vi "xeva-main.vi"() -> ()   [LabVIEW 2015]
uses:
  <vilib>/Xenics Infrared Solutions/Xeneth LabVIEW API/Xeneth.lvlib
panel:
  in  "stop-acquisition":bool
  out "Histogram":T1(graph)={"X Values"=[381.555, 1026.665, 1671.775, 2316.885, 2961.995, 3607.105, 4252.215, 4897.325, 5542.435, 6187.545, 6832.655, 7477.765, 8122.875, 8767.985, 9413.095, 10058.205, 10703.315, 11348.425, 11993.535, 12638.645, 13283.755, 13928.865, 14573.975, 15219.085, 15864.195, 16509.305, 17154.415, 17799.525, 18444.635, 19089.745, 19734.855, 20379.965, 21025.075, 21670.185, 22315.295, 22960.405, 23605.515, 24250.625, 24895.735, 25540.845, 26185.955, 26831.065, 27476.175, 28121.285, 28766.395, 29411.505, 30056.615, 30701.725, 31346.835, 31991.945, 32637.055, 33282.165, 33927.275, 34572.385, 35217.495, 35862.605, 36507.715, 37152.825, 37797.935, 38443.045, 39088.155, 39733.265, 40378.375, 41023.485, 41668.595, 42313.705, 42958.815, 43603.925, 44249.035, 44894.145, 45539.255, 46184.365, 46829.475, 47474.585, 48119.695, 48764.805, 49409.915, 50055.025, 50700.135, 51345.245, 51990.355, 52635.465, 53280.575, 53925.685, 54570.795, 55215.905, 55861.015, 56506.125, 57151.235, 57796.345, 58441.455, 59086.565, 59731.675, 60376.785, 61021.895, 61667.005, 62312.115, 62957.225, 63602.335, 64247.445], "Histogram: h(x)"=[235, 173, 0, 115, 75, 0, 36, 38, 0, 21, 0, 14, 13, 0, 16, 28, 0, 49, 0, 91, 118, 0, 184, 328, 0, 436, 626, 0, 854, 0, 1158, 1443, 0, 1891, 2217, 0, 2808, 0, 3354, 3711, 0, 4252, 4588, 0, 4786, 0, 4898, 4792, 0, 4596, 4273, 0, 3970, 3545, 0, 3221, 0, 3015, 2668, 0, 2533, 2324, 0, 2214, 0, 2124, 1991, 0, 1897, 1839, 0, 1906, 0, 1861, 1832, 0, 1883, 1841, 0, 1844, 1875, 0, 1813, 0, 1765, 1729, 0, 1611, 1524, 0, 1290, 0, 1154, 968, 0, 749, 585, 0, 491, 313]}
  out "data":u16[][](array[numeric])
  out "error out":errorcluster
  out "temperature reached":bool
  in  "stop-parameter-read":bool
  out "cooling":bool
  out "temperature":bool
  in  "temperature / °C":dbl=-10.0
  out "Parameter":T2 {"time" format="%#.2g"}
  out "integration time":bool
  in  "integration time / s":dbl=1.0
  out "xeva initialized":bool
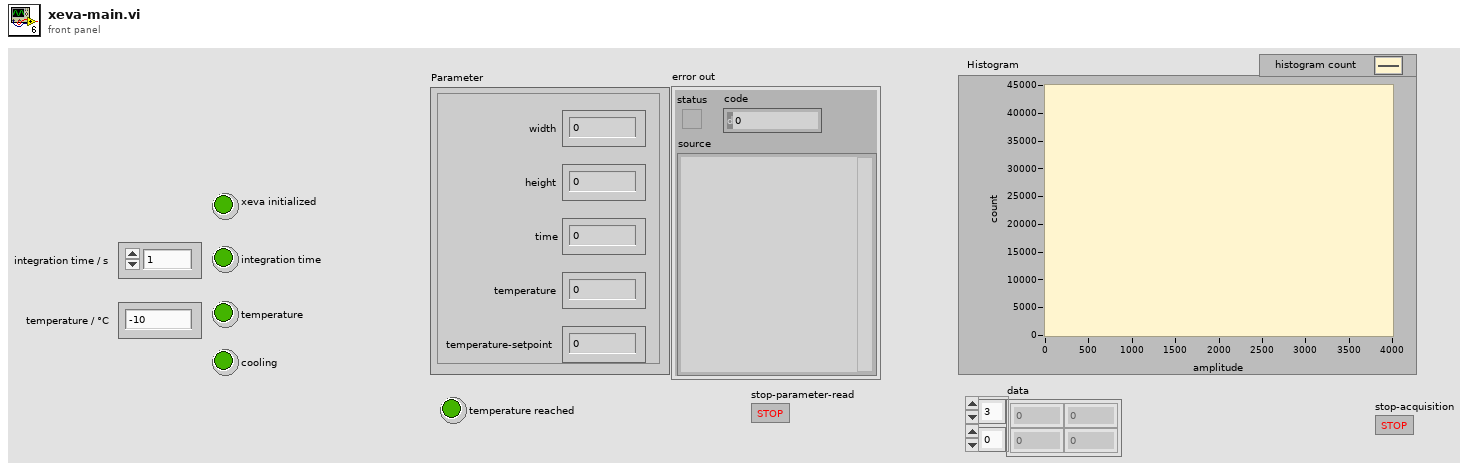
[diagram p1: front panel]
types:
  T1 = cluster{"X Values":dbl[], "Histogram: h(x)":i32[]}
  T2 = cluster{"width":u32, "height":u32, "time":dbl, "temperature":dbl, "temperature-setpoint":dbl}
  T3 = typedef "Xeneth.lvlib/Camara.ctl" = refnum<k1>
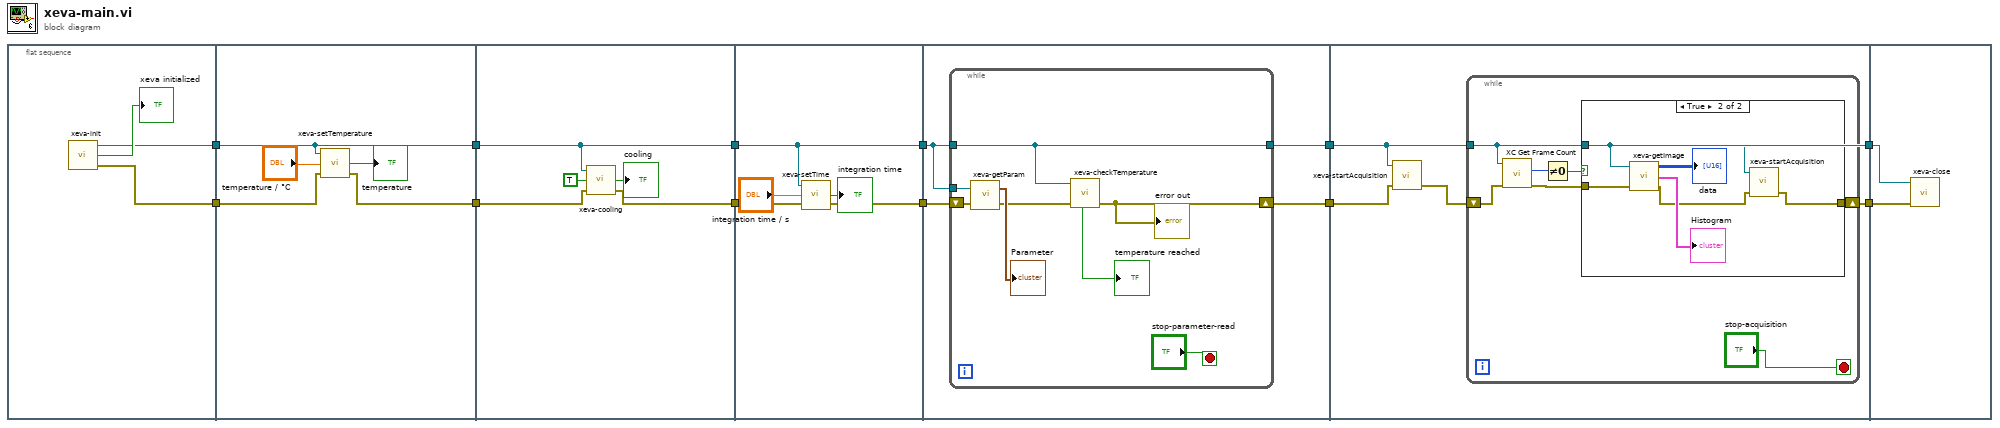
[diagram p0: block diagram]
diagram:
  n1 = flat-sequence {
    tunnel: [w14] -> w10
    tunnel: [w13] -> w9
    tunnel: w10 -> [w18]
    tunnel: [w18] -> w8
    tunnel: w9 -> [w20]
    tunnel: [w19] -> w6
    tunnel: w8 -> [w23]
    tunnel: [w23] -> w7
    tunnel: w6 -> [w25]
    tunnel: [w24] -> w5
    tunnel: w7 -> [w28]
    tunnel: [w28] -> w12
    tunnel: w5 -> [w29]
    tunnel: [w30] -> w11
    tunnel: w12 -> [w32]
    tunnel: [w31] -> w4
    tunnel: [w33] -> w2
    tunnel: w11 -> [w34]
    tunnel: w4 -> [w43]
    tunnel: [w43] -> w3
    tunnel: w2 -> [w46]
    tunnel: [w45] -> w1
    tunnel: w3 -> [w62]
    tunnel: w1 -> [w61]
    frame #0 {
      n2 = call "xeva-init.vi"() -> ("error out"=w13:errorcluster, "initialized"=→"xeva initialized":bool, "xeva-camref"=w14:T3)  [unwired: 3 in]
    }
    frame #1 {
      n3 = call "xeva-setTemperature.vi"("error in (no error)"=w20, "xeva-temperature"="temperature / °C", "xeva-camref"=w18) -> ("error out"=w19:errorcluster, "xeva-temperatureSP-ok"=→"temperature":bool)  [unwired: 1 in]
    }
    frame #2 {
      n4 = call "xeva-cooling.vi"("error in (no error)"=w25, "xeva-cool-on"=TRUE ("xeneth-cool"), "xeva-camref"=w23) -> ("error out"=w24:errorcluster, "xeva-cooling"=→"cooling":bool)  [unwired: 1 in]
    }
    frame #3 {
      n5 = call "xeva-setTime.vi"("error in (no error)"=w29, "xeva-time"="integration time / s", "xeva-camref"=w28) -> ("error out"=w30:errorcluster, "xeva-time-ok"=→"integration time":bool)  [unwired: 1 in]
    }
    frame #4 {
      n6 = while {
        tunnel: w32 -> [w40]
        shift-right: [w35] -> w33
        shift-left: w34 -> [w42]
        tunnel: w32 -> [w37]
        tunnel: [w37] -> w31
        stop <- "stop-parameter-read" stop-if-true
        n7 = call "xeva-getParam.vi"("error in (no error)"=w42, "xeva-camref"=w40) -> ("error out"=w38:errorcluster, "xeva-parameters"=→"Parameter":T2)
        n8 = call "xeva-checkTemperature.vi"("error in (no error)"=w38, "xeva-camref"=w37) -> ("error out"=w35:errorcluster, "xeva-temperature-reached"=→"temperature reached":bool)  [unwired: 2 in]
        "error out" <- w35
      }
    }
    frame #5 {
      n9 = call "xeva-startAcquisition.vi"("error in (no error)"=w46, "xeva-camref"=w43) -> ("error out"=w44:errorcluster)  [unwired: 1 in, 2 out]
      n10 = while {
        tunnel: w43 -> [w51]
        shift-right: [w53] -> w45
        shift-left: w44 -> [w52]
        stop <- "stop-acquisition" stop-if-true
        n11 = call <vilib>:"XC Get Frame Count.vi"("error in (no error)"=w52, "Cam Ref"=w51) -> ("error out"=w48:errorcluster, "Frame Count"=w50:u32)  [unwired: 7 in, 1 out]
        n12 = Not Equal To 0?(x=w50) -> (x != 0?=w49:bool)
        n13 = case shown="True" w49 {
          tunnel: [w54 w56] -> w53
          tunnel: w51 -> [_ w55]
          tunnel: w48 -> [w54 w58]
          frame False {
          }
          frame True {
            n14 = call "xeva-getImage.vi"("error in (no error)"=w58, "xeva-camref"=w55) -> ("error out"=w57:errorcluster, "xeva-histogram"=→"Histogram":T1, "xeva-data"=→"data":u16[][])  [unwired: 1 in]
            n15 = call "xeva-startAcquisition.vi"("error in (no error)"=w57, "xeva-camref"=w55) -> ("error out"=w56:errorcluster)  [unwired: 1 in, 2 out]
          }
        }
      }
    }
    frame #6 {
      n16 = call "xeva-close.vi"("error in (no error)"=w61, "xeva-camref"=w62) -> ()  [unwired: 3 in, 1 out]
    }
  }
